vi "Update Stiffness Jacobian.vi"(6 "Stiffness Limit":dbl[][](array[numeric]), 9 "Mixed Mode Convergence Status In":T3, 10 "Increments":T5, 11 "Stiffness Jacobian In":T4=[[1000000.0, 0.0, 0.0, 0.0, 0.0, 0.0], [0.0, 1000000.0, 0.0, 0.0, 0.0, 0.0], [0.0, 0.0, 1000000.0, 0.0, 0.0, 0.0], [0.0, 0.0, 0.0, 1000000.0, 0.0, 0.0], [0.0, 0.0, 0.0, 0.0, 1000000.0, 0.0], [0.0, 0.0, 0.0, 0.0, 0.0, 1000000.0]]) -> (1 "Jacobian Stiffness Column":T1, 3 "Stiffness Jacobian Out":T4=[[1000000.0, 0.0, 0.0, 0.0, 0.0, 0.0], [0.0, 1000000.0, 0.0, 0.0, 0.0, 0.0], [0.0, 0.0, 1000000.0, 0.0, 0.0, 0.0], [0.0, 0.0, 0.0, 1000000.0, 0.0, 0.0], [0.0, 0.0, 0.0, 0.0, 1000000.0, 0.0], [0.0, 0.0, 0.0, 0.0, 0.0, 1000000.0]])   [LabVIEW 2009]
uses:
  Mixed Mode Cartesian Data.ctl
  Stiffness Matrix.ctl
  Mixed Mode Convergence Status.ctl
  Global Data/Jacobian Stiffness Column.ctl
  Global Data/Jacobian Stiffness Column Id.ctl
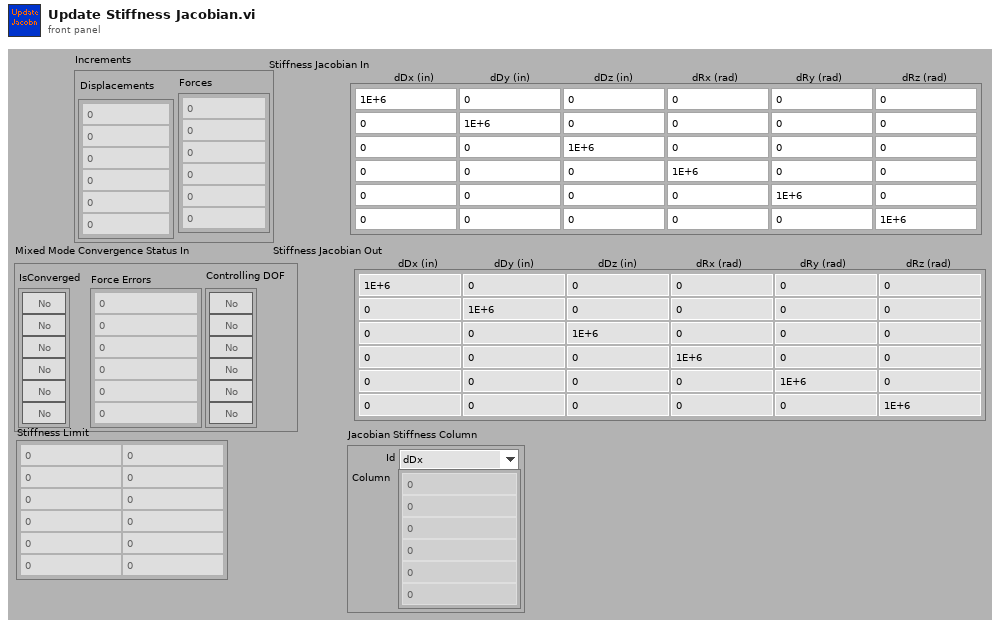
[diagram p1: front panel]
types:
  T1 = typedef "Jacobian Stiffness Column.ctl" = cluster{"Id":T2, "Column":dbl[]}
  T2 = typedef "Jacobian Stiffness Column Id.ctl" = enum16{"dDx", "dDy", "dDz", "dRx", "dRy", "dRz"}
  T3 = typedef "Mixed Mode Convergence Status.ctl" = cluster{"IsConverged":bool[], "Force Errors":dbl[], "Controlling DOF":bool[]}
  T4 = typedef "Stiffness Matrix.ctl" = dbl[][]
  T5 = typedef "Mixed Mode Cartesian Data.ctl" = cluster{"Displacements":dbl[], "Forces":dbl[]}
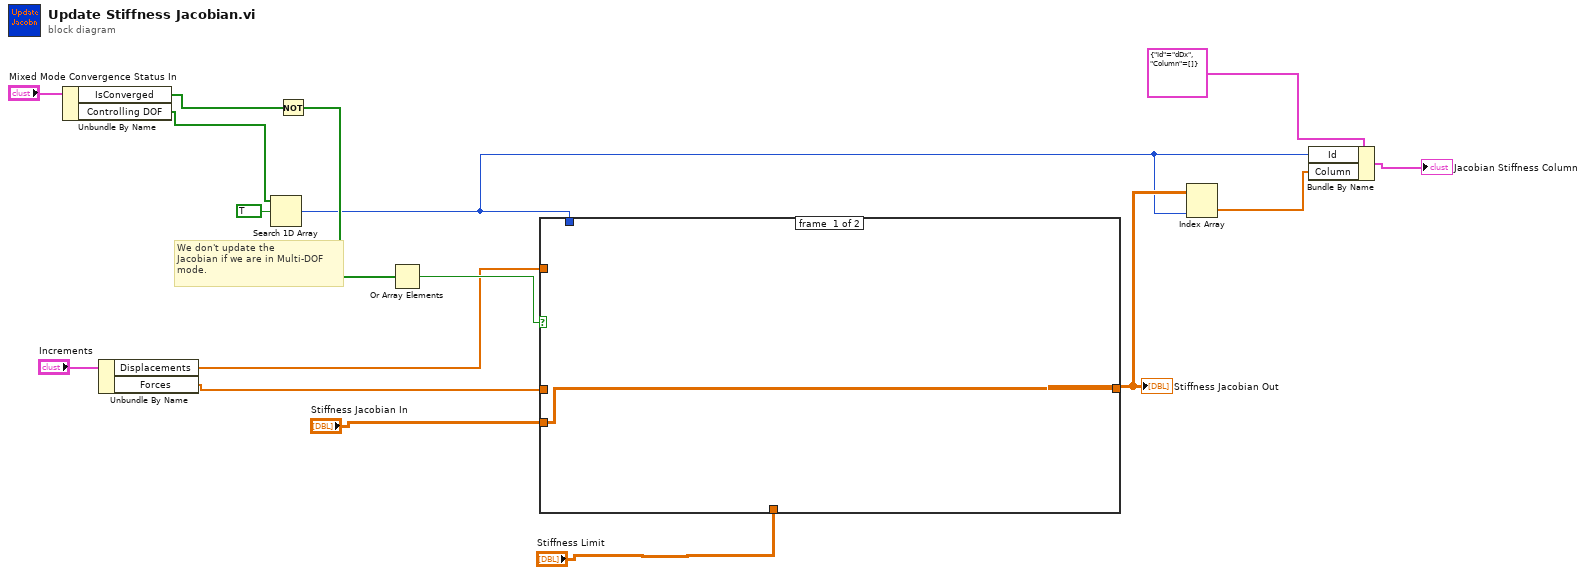
[diagram p0: block diagram]
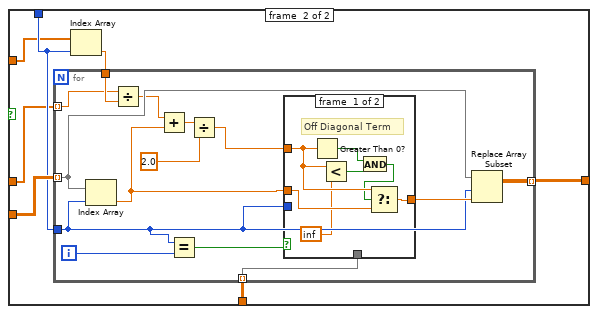
[diagram p2: hidden frame]
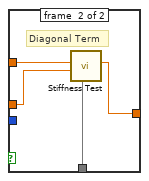
[diagram p3: hidden frame]
diagram:
  # "We don't update the \nJacobian if we are in Multi-DOF\nmode."
  n1 = Unbundle By Name("Mixed Mode Convergence Status In") -> ("IsConverged"=w10:bool[], "Controlling DOF"=w8:bool[])
  n2 = Unbundle By Name("Increments") -> ("Displacements"=w12:dbl[], "Forces"=w14:dbl[])
  n3 = Search 1D Array(1D array=w8, element=TRUE) -> (index of element=w2:i32)  [unwired: 1 in]
  n4 = Not(x=w10) -> (.not. x?=w9:bool[])
  n5 = Or Array Elements(Boolean array=w9) -> (logical OR=w13:bool)
  n6 = case shown="True" w13 {
    tunnel: "Stiffness Jacobian In" -> [w17 w24]
    tunnel: w2 -> [_ w23]
    tunnel: w14 -> [_ w22]
    tunnel: [w17 w20] -> w3
    tunnel: w12 -> [_ w19]
    tunnel: "Stiffness Limit" -> [_ w18]
    frame #0 {
    }
    frame #1 {
      n7 = Index Array(array=w19, index=w23) -> (element=w21:dbl)
      n8 = for {
        tunnel: w24 -> [w37] mode=indexing
        tunnel: w23 -> [w28]
        tunnel: w22 -> [w35] mode=indexing
        tunnel: w21 -> [w38]
        tunnel: [w36] -> w20 mode=indexing
        tunnel: w18 -> [w29] mode=indexing
        i -> [w27]
        n9 = Index Array(array=w37, index=w28) -> (element=w25:dbl)
        n10 = Divide(x=w35, y=w38) -> (x/y=w34:dbl)
        n11 = Add(x=w34, y=w25) -> (x+y=w33:dbl)
        n12 = Equal?(x=w28, y=w27) -> (x = y?=w26:bool)
        n13 = Divide(x=w33, y=2.0) -> (x/y=w31:dbl)
        n14 = case shown="True" w26 {
          tunnel: w31 -> [w42 w49]
          tunnel: [w45 w48] -> w30
          tunnel: w29 -> [_ w47]
          tunnel: w28 -> [_ _]
          tunnel: w25 -> [w43 w46]
          frame #0 {
            # "Off Diagonal Term"
            n15 = Greater Than 0?(x=w42) -> (x > 0?=w44:bool)
            n16 = Less?(x=w42, y=inf) -> (x < y?=w39:bool)
            n17 = And(x=w44, y=w39) -> (x .and. y?=w40:bool)
            n18 = Select(t=w42, s=w40, f=w43) -> (s? t:f=w45:dbl)
          }
          frame #1 {
            # "Diagonal Term"
            n19 = call "Stiffness Test.vi"("Limits"=w47, "Prev Stiffness Value"=w46, "Stiffness Value In"=w49) -> ("Stiffness Value Out"=w48:dbl)  [unwired: 8 in]
          }
        }
        n20 = Replace Array Subset(array=w37, new element=w30, index=w28) -> (w36:dbl[])
      }
    }
  }
  "Stiffness Jacobian Out" <- w3
  n21 = Index Array(array=w3, index (col)=w2) -> (element=w1:dbl[])  [unwired: 1 in]
  n22 = Bundle By Name(cluster=T1 {"Id"=enum."dDx", "Column"=[]} ("Jacobian Stiffness Column"), "Id"=w2, "Column"=w1) -> (→"Jacobian Stiffness Column":T1)
